vi "2exp fit.vi"(8 "y":dbl[](array[numeric]) format="%.2f", 9 "x":dbl[](array[numeric]) format="%.2f") -> (1 "Best Fit":dbl[](array[numeric]), 2 "off":dbl format="%.3f", 3 "on":dbl format="%.3f")   [LabVIEW 2009]
panel:
  in  "n: fit-channels 2":i32=600
  out "on 3":dbl format="%.2f"
  out "off 3":dbl format="%.2f"
  out "ac":dbl format="%.2f"
  in  "S+B":dbl format="%.2f"
  in  "B":dbl=500.0 format="%.2f"
  out "A measured":dbl format="%.2f"
  out "A corrected":dbl format="%.2f"
  in  "biexpo fit?":bool=TRUE
  out "ac 2":dbl format="%.2f"
  out "off 2":dbl format="%.3f"
  out "on 2":dbl format="%.3f"
  out "A corrected 2":dbl format="%.2f"
  out "element":dbl format="%.2f"
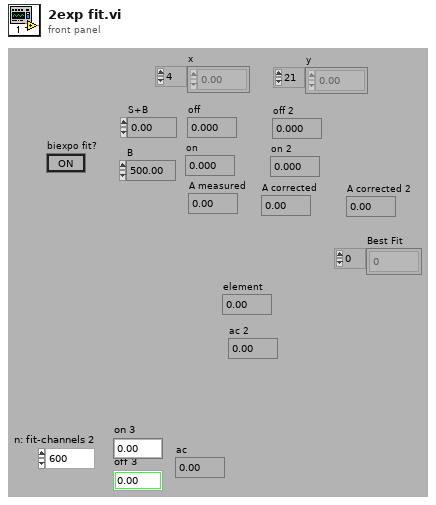
[diagram p1: front panel]
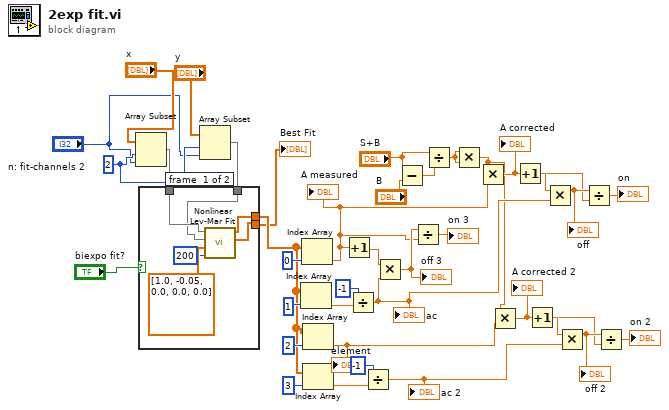
[diagram p0: block diagram]
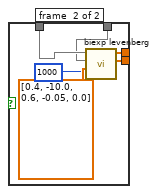
[diagram p2: hidden frame]
diagram:
  w3 = 2 ("Array Index")
  n1 = Array Subset(array="x", index=w3, length="n: fit-channels 2") -> (w20:dbl[])
  n2 = Array Subset(array="y", index=w3, length="n: fit-channels 2") -> (w1:dbl[])
  n3 = case shown="False" "biexpo fit?" {
    tunnel: w20 -> [w39 w45]
    tunnel: [w41 w48] -> w14
    tunnel: [w40 w47] -> w5
    tunnel: w1 -> [w38 w44]
    frame #0 {
      n4 = call "Nonlinear Lev-Mar Fit.vi"("max iteration"=200, "Initial Guess Coefficients"=dbl[] [1.0, -0.05, 0.0, 0.0, 0.0] ("Guess Coefficients 2"), "Y"=w38, "X"=w39) -> ("Best Fit"=w40:dbl[], "Best Fit Coefficients"=w41:dbl[])  [unwired: 2 in, 3 out]
    }
    frame #1 {
      n5 = call "biexp levenberg.vi"("max iteration"=1000, "Initial Guess Coefficients"=dbl[] [0.4, -10.0, 0.6, -0.05, 0.0], "Y"=w44, "X"=w45) -> ("Best Fit"=w47:dbl[], "Best Fit Coefficients"=w48:dbl[])  [unwired: 2 in, 3 out]
    }
  }
  "Best Fit" <- w5
  n6 = Index Array(array=w14, index=1 ("Index")) -> (element=w31:dbl)
  n7 = Index Array(array=w14, index=0 ("Index")) -> (element=w22:dbl)
  "A measured" <- w22
  n8 = Index Array(array=w14, index=2) -> (element=w8:dbl)
  "element" <- w8
  n9 = Index Array(array=w14, index=3) -> (element=w15:dbl)
  n10 = Increment(x=w22) -> (x+1=w37:dbl)
  n11 = Divide(x=-1 ("Array Index"), y=w31) -> (x/y=w25:dbl)
  "ac" <- w25
  n12 = Divide(x=-1 ("Array Index"), y=w15) -> (x/y=w7:dbl)
  "ac 2" <- w7
  n13 = Multiply(x=w37, y=w25) -> (x*y=w33:dbl)
  "off 3" <- w33
  n14 = Subtract(x="S+B", y="B") -> (x-y=w28:dbl)
  n15 = Divide(x=w33, y=w22) -> (x/y=→"on 3":dbl)
  n16 = Divide(x="S+B", y=w28) -> (x/y=w27:dbl)
  n17 = Multiply(x=w27, y=w27) -> (x*y=w9:dbl)
  n18 = Multiply(x=w9, y=w22) -> (x*y=w21:dbl)
  "A corrected" <- w21
  n19 = Multiply(x=w9, y=w8) -> (x*y=w10:dbl)
  "A corrected 2" <- w10
  n20 = Increment(x=w21) -> (x+1=w26:dbl)
  n21 = Increment(x=w10) -> (x+1=w13:dbl)
  n22 = Multiply(x=w26, y=w25) -> (x*y=w24:dbl)
  "off" <- w24
  n23 = Multiply(x=w13, y=w7) -> (x*y=w12:dbl)
  "off 2" <- w12
  n24 = Divide(x=w24, y=w21) -> (x/y=→"on":dbl)
  n25 = Divide(x=w12, y=w10) -> (x/y=→"on 2":dbl)
